vi "mecanum_calc.vi"(11 "Command":T2) -> (3 "Ouput":T1)   [LabVIEW 2012]
uses:
  mecanum_control.ctl
  mecanum_output.ctl
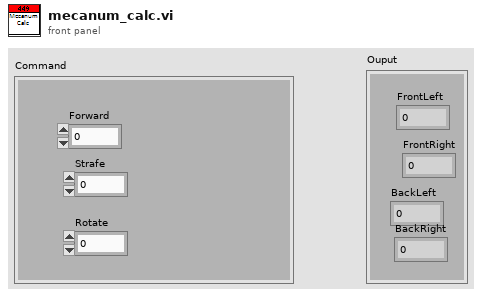
[diagram p1: front panel]
types:
  T1 = typedef "mecanum_output.ctl" = cluster{"FrontLeft":dbl, "FrontRight":dbl, "BackLeft":dbl, "BackRight":dbl}
  T2 = typedef "mecanum_control.ctl" = cluster{"Forward":dbl, "Strafe":dbl, "Rotate":dbl}
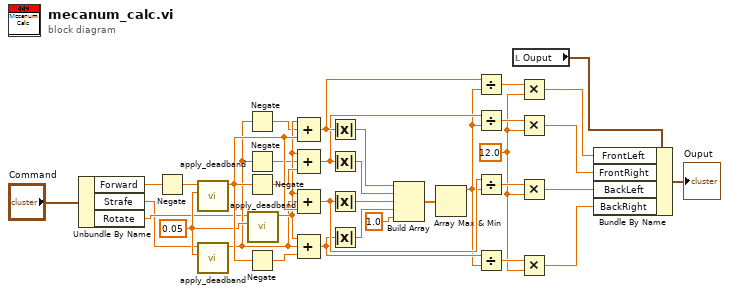
[diagram p0: block diagram]
diagram:
  w15 = 0.05
  w19 = 12.0 ("y")
  n1 = Unbundle By Name("Command") -> ("Forward"=w7:dbl, "Strafe"=w8:dbl, "Rotate"=w9:dbl)
  n2 = Negate(x=w7) -> (-x=w14:dbl)
  n3 = call "apply_deadband.vi"("Deadband"=w15, "Input"=w14) -> ("Input with deadband"=w17:dbl)  [unwired: 9 in]
  n4 = call "apply_deadband.vi"("Deadband"=w15, "Input"=w8) -> ("Input with deadband"=w13:dbl)  [unwired: 9 in]
  n5 = Negate(x=w13) -> (-x=w12:dbl)
  n6 = Negate(x=w13) -> (-x=w11:dbl)
  n7 = Negate(x=w17) -> (-x=w35:dbl)
  n8 = Negate(x=w17) -> (-x=w34:dbl)
  n9 = call "apply_deadband.vi"("Deadband"=w15, "Input"=w9) -> ("Input with deadband"=w16:dbl)  [unwired: 9 in]
  n10 = Compound Arithmetic op=ADD(w16, w12, w17) -> (w29:dbl)
  n11 = Compound Arithmetic op=ADD(w16, w11, w35) -> (w25:dbl)
  n12 = Compound Arithmetic op=ADD(w16, w13, w17) -> (w24:dbl)
  n13 = Compound Arithmetic op=ADD(w16, w13, w34) -> (w22:dbl)
  n14 = Absolute Value(x=w29) -> (abs(x)=w33:dbl)
  n15 = Absolute Value(x=w25) -> (abs(x)=w28:dbl)
  n16 = Absolute Value(x=w24) -> (abs(x)=w32:dbl)
  n17 = Absolute Value(x=w22) -> (abs(x)=w31:dbl)
  n18 = Build Array(w33, w28, w32, w31, 1.0 ("element")) -> (w30:dbl[])
  n19 = Array Max & Min(array=w30) -> (max value=w21:dbl)  [unwired: 3 out]
  n20 = Divide(x=w29, y=w21) -> (x/y=w26:dbl)
  n21 = Divide(x=w25, y=w21) -> (x/y=w27:dbl)
  n22 = Divide(x=w24, y=w21) -> (x/y=w23:dbl)
  n23 = Divide(x=w22, y=w21) -> (x/y=w20:dbl)
  n24 = local read "Ouput"() -> (w6:T1)
  n25 = Multiply(x=w26, y=w19) -> (x*y=w3:dbl)
  n26 = Multiply(x=w27, y=w19) -> (x*y=w1:dbl)
  n27 = Multiply(x=w23, y=w19) -> (x*y=w2:dbl)
  n28 = Multiply(x=w20, y=w19) -> (x*y=w4:dbl)
  n29 = Bundle By Name(cluster=w6, "FrontLeft"=w3, "FrontRight"=w1, "BackLeft"=w2, "BackRight"=w4) -> (→"Ouput":T1)
